vi "MainVI.vi"(0 "VISA resource name":refnum<visa-resource-name>="COM11", 1 "baud rate":u32=115200, 2 "data bits":u16=8 min=5 max=8 step=1, 3 "parity":u16(ring) items=["None", "Odd", "Even", "Mark", "Space"], 4 "stop bits":u16(ring)=10 items=["1.0"=10, "1.5"=15, "2.0"=20], 6 "read":bool=TRUE, 7 "flow control":u16(ring) items=["None"=0, "XON/XOFF"=1, "RTS/CTS"=2, "DTR/DSR"=4]) -> (9 "read string":string, 10 "bytes read":u32)   [LabVIEW 2017]
doc: "The Basic Serial Read and Write example performs a Serial Port Read, a Serial Port Write, or a combination of these actions. The user selects the actions (read or write) on the front panel. If both are selected, the VI will write the data first, read data, and then close the VISA session that is opened to the port. This VI will wait until the specified number of bytes is received at the port. Only the number of bytes specified will be read.\n\nINSTRUCTIONS:\n1) Select the serial resource and configuration parameters (baud rate, data bits, parity, stop bits, flow control).\n2) Select the operations to be performed. \n3) Connect the serial port to your device. If no device is available, perform a loopback test by doing one of the following. Short pins 2 and 3 on a RS-232 cable or short pin 4 to pin 8 and pin 5 to pin 9 on a RS-485/422 cable. \n4) Run the VI to see the data read. (The \"read string\" will match the \"string to write\" if a loopback test was performed.)\n\nNote: The parameters set for the serial port must match the parameters of the connected instrument or device. In this example, the bytes to read parameter specifies the number of bytes that the serial port reads. If there were more bytes at the port than the number specified in bytes to read, those bytes would not be read. Also, if you specify to read more bytes than the number of bytes actually read, you might receive a timeout error message.\n\nOn the block diagram, the Configure Serial Port VI sets the configuration parameters. The front panel displays the controls used to configure the basic parameters, such as baud rate, data bits, and parity. Constants configure the other parameters the user probably does not need set. After the VISA Configure Serial Port VI opens the VISA session and configures the port, the VI passes the VISA resource name to other VIs that perform operations on that VISA resource. The VISA Write function sends a command to the serial device and the VISA Read function returns data based on the command. The VISA Close function then closes the reference to the serial device. It is important to close the reference; otherwise communication through with that port through protocols other than VISA might not be possible."
uses:
  <vilib>/ErrorRing/Error Ring.xnode
panel:
  in  "file path (dialog if empty)":path
  in  "Tab Control":enum32{"Main", "Terminal", "Connect"}(tab)=enum."Terminal"
  out "Waveform Chart 4":dbl(graph)
  out "Waveform Chart 3":dbl(graph)
  out "Waveform Chart 2":dbl(graph)
  out "Waveform Chart":dbl(graph)
  in  "DTC":bool
  in  "Engine load":bool
  in  "Coolant temp.":bool
  in  "Engine RPM":bool
  in  "Speed":bool
  in  "Save to file":bool
  in  "Repeat":bool
  out "Return Count":u32
  in  "write":bool
  in  "string to write":string="ATZ"
  in  "Connect":bool
  in  "wbc":dbl=4.0
  out "Succses":u32
  in  "delay before read (ms)":u32=265
  out "Status":bool
  out "error out":errorcluster
  in  "stop":bool
  in  "Cancel Button":bool
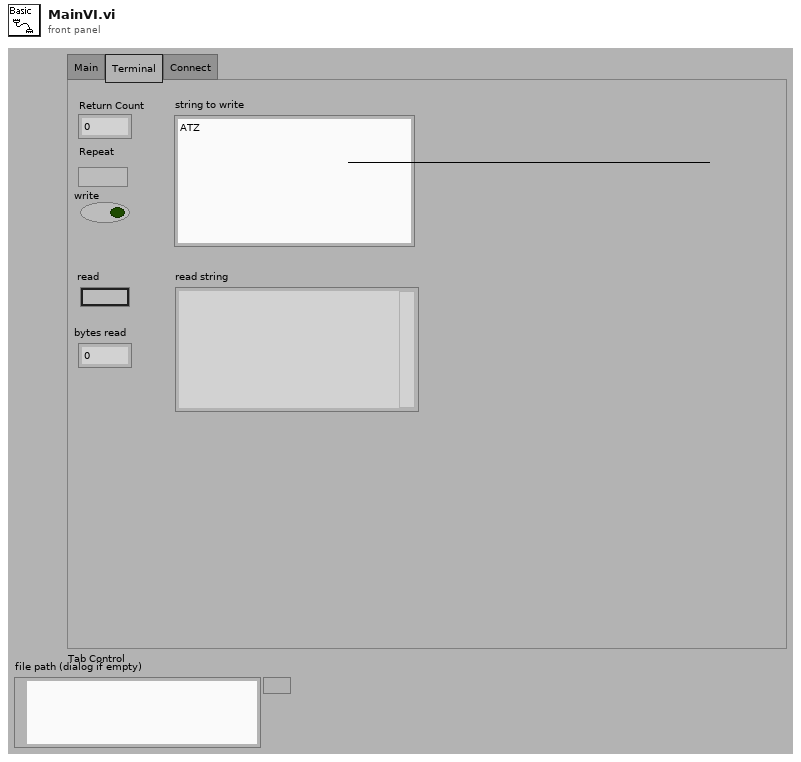
[diagram p1: front panel]
types:
  T1 = enum16{"open", "replace", "create", "open or create", "replace or create", "replace or create with confirmation"}
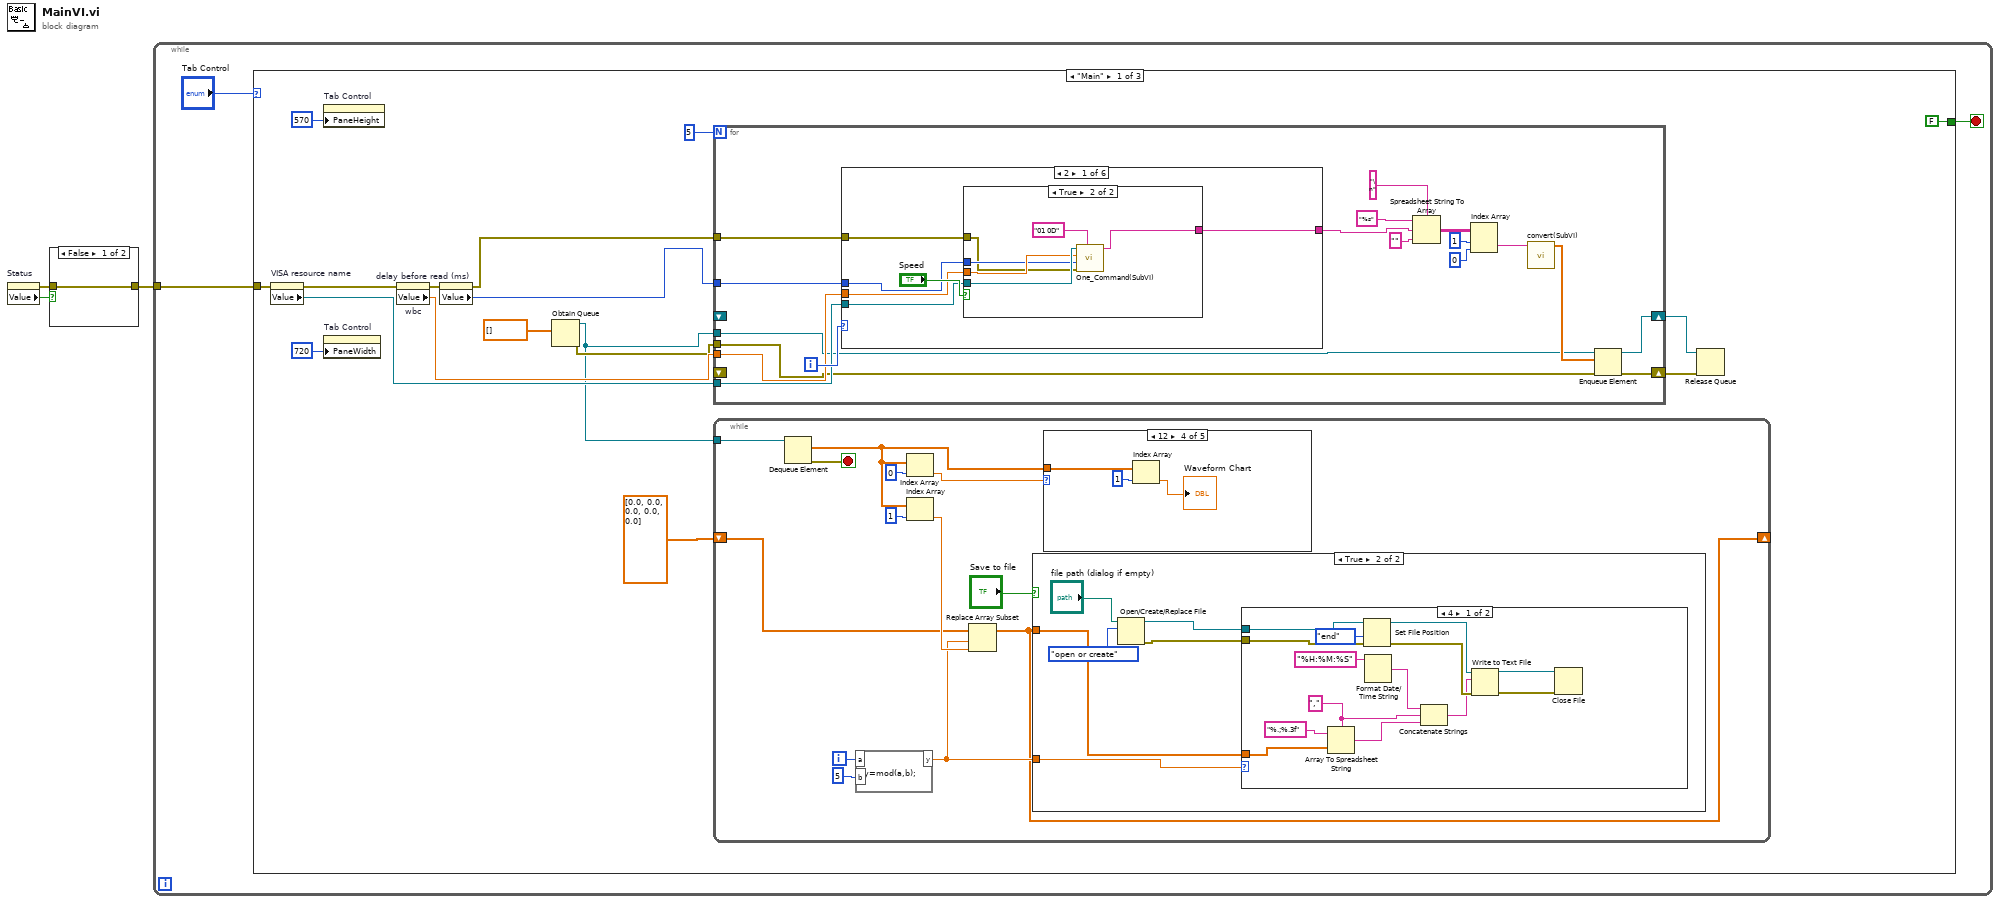
[diagram p0: block diagram]
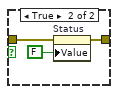
[diagram p2: hidden frame]
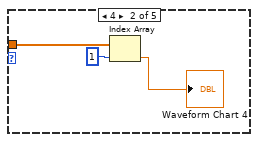
[diagram p6: hidden frame]
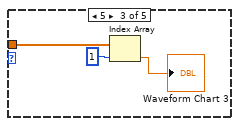
[diagram p7: hidden frame]
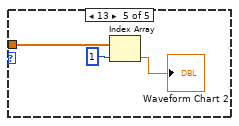
[diagram p8: hidden frame]
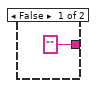
[diagram p9: hidden frame]
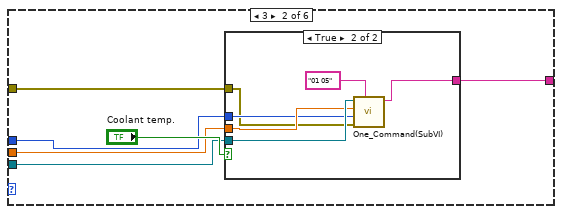
[diagram p10: hidden frame]
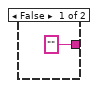
[diagram p11: hidden frame]
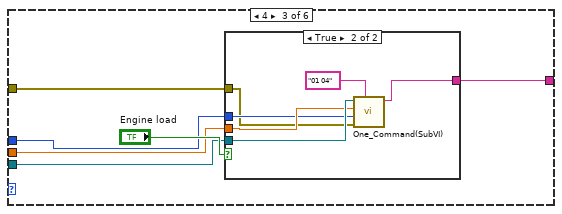
[diagram p12: hidden frame]
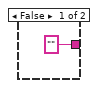
[diagram p13: hidden frame]
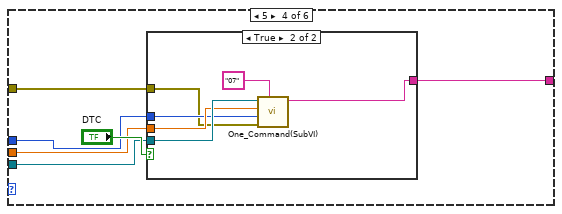
[diagram p14: hidden frame]
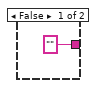
[diagram p15: hidden frame]
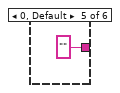
[diagram p16: hidden frame]
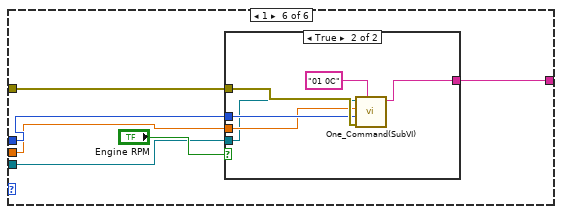
[diagram p17: hidden frame]
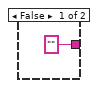
[diagram p18: hidden frame]
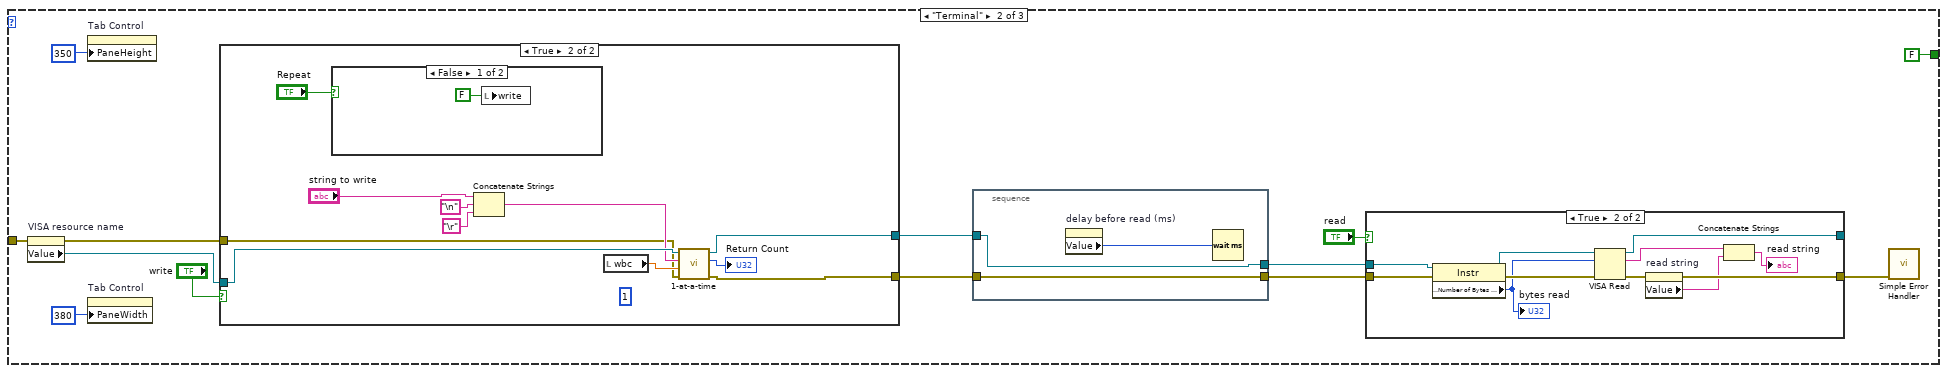
[diagram p19: hidden frame]
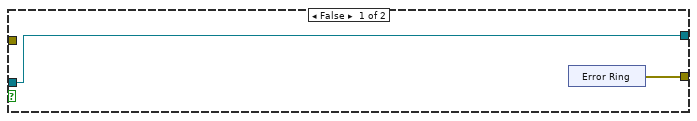
[diagram p20: hidden frame]
diagram:
  n1 = property on="Status" class="Bool (strict)"() -> (error out=w3:errorcluster, "Value"=w2:bool)  [unwired: 2 in, 1 out]
  n2 = case shown="False" w2 {
    tunnel: [w4 w7] -> w1
    tunnel: w3 -> [w4 w5]
    frame False {
    }
    frame True {
      n3 = property on="Status" class="Bool (strict)"(error in=w5, "Value"=FALSE) -> (error out=w7:errorcluster)  [unwired: 1 in, 1 out]
    }
  }
  n4 = while {
    tunnel: w1 -> [w8]
    stop <- w9 stop-if-true
    n5 = case shown="\"Main\"" "Tab Control" {
      tunnel: [FALSE FALSE "Cancel Button"] -> w9
      tunnel: w8 -> [w23 w157 w201]
      frame "Main" {
        n6 = property on="VISA resource name" class="VISAName"(error in=w23) -> (error out=w22:errorcluster, "Value"=w19:refnum<visa-resource-name>)  [unwired: 1 in, 1 out]
        n7 = property on="Tab Control" class="TabCtl (strict)"("PaneHeight"=570) -> ()  [unwired: 2 in, 2 out]
        n8 = property on="Tab Control" class="TabCtl (strict)"("PaneWidth"=720) -> ()  [unwired: 2 in, 2 out]
        n9 = property on="wbc" class="DigNum (strict)"(error in=w22) -> (error out=w21:errorcluster, "Value"=w18:dbl)  [unwired: 1 in, 1 out]
        n10 = property on="delay before read (ms)" class="DigNum (strict)"(error in=w21) -> (error out=w20:errorcluster, "Value"=w17:u32)  [unwired: 1 in, 1 out]
        n11 = Obtain Queue(element data type=dbl[] []) -> (queue out=w12:refnum<queue>, error out=w15:errorcluster)  [unwired: 4 in, 1 out]
        n12 = for {
          N: 5 -> [_]
          tunnel: w20 -> [w89]
          tunnel: w19 -> [w86]
          tunnel: w18 -> [w87]
          tunnel: w17 -> [w88]
          tunnel: w12 -> [w76]
          tunnel: w15 -> [w75]
          shift-right: [w74] -> w14
          shift-left: _ -> [_]
          shift-right: [w73] -> w13
          shift-left: _ -> [_]
          i -> [w90]
          n13 = case shown="2" w90 {
            tunnel: w89 -> [w95 w108 w121 w134 _ w148]
            tunnel: w88 -> [w92 w105 w118 w131 _ w147]
            tunnel: w87 -> [w93 w106 w119 w132 _ w146]
            tunnel: w86 -> [w94 w107 w120 w133 _ w145]
            tunnel: [w91 w104 w117 w130 "" w144] -> w82
            frame 2 {
              n14 = case shown="True" "Speed" {
                tunnel: w95 -> [_ w100]
                tunnel: w94 -> [_ w103]
                tunnel: w93 -> [_ w102]
                tunnel: w92 -> [_ w101]
                tunnel: ["" w98] -> w91
                frame False {
                }
                frame True {
                  n15 = call "One_Command(SubVI).vi"("string to write"="01 0D", "error in (no error)"=w100, "delay before read (ms)"=w101, "wbc"=w102, "VISA resource name"=w103) -> ("read string"=w98:string)  [unwired: 5 in, 1 out]
                }
              }
            }
            frame 3 {
              n16 = case shown="True" "Coolant temp." {
                tunnel: w108 -> [_ w113]
                tunnel: w107 -> [_ w116]
                tunnel: w106 -> [_ w115]
                tunnel: w105 -> [_ w114]
                tunnel: ["" w111] -> w104
                frame False {
                }
                frame True {
                  n17 = call "One_Command(SubVI).vi"("string to write"="01 05", "error in (no error)"=w113, "delay before read (ms)"=w114, "wbc"=w115, "VISA resource name"=w116) -> ("read string"=w111:string)  [unwired: 5 in, 1 out]
                }
              }
            }
            frame 4 {
              n18 = case shown="True" "Engine load" {
                tunnel: w121 -> [_ w126]
                tunnel: w120 -> [_ w129]
                tunnel: w119 -> [_ w128]
                tunnel: w118 -> [_ w127]
                tunnel: ["" w124] -> w117
                frame False {
                }
                frame True {
                  n19 = call "One_Command(SubVI).vi"("string to write"="01 04", "error in (no error)"=w126, "delay before read (ms)"=w127, "wbc"=w128, "VISA resource name"=w129) -> ("read string"=w124:string)  [unwired: 5 in, 1 out]
                }
              }
            }
            frame 5 {
              n20 = case shown="True" "DTC" {
                tunnel: w134 -> [_ w138]
                tunnel: w133 -> [_ w141]
                tunnel: w132 -> [_ w140]
                tunnel: w131 -> [_ w139]
                tunnel: ["" w137] -> w130
                frame False {
                }
                frame True {
                  n21 = call "One_Command(SubVI).vi"("string to write"="07", "error in (no error)"=w138, "delay before read (ms)"=w139, "wbc"=w140, "VISA resource name"=w141) -> ("read string"=w137:string)  [unwired: 5 in, 1 out]
                }
              }
            }
            frame 0, Default {
            }
            frame 1 {
              n22 = case shown="True" "Engine RPM" {
                tunnel: w148 -> [_ w156]
                tunnel: w147 -> [_ w155]
                tunnel: w146 -> [_ w154]
                tunnel: w145 -> [_ w153]
                tunnel: ["" w151] -> w144
                frame False {
                }
                frame True {
                  n23 = call "One_Command(SubVI).vi"("string to write"="01 0C", "error in (no error)"=w156, "delay before read (ms)"=w155, "wbc"=w154, "VISA resource name"=w153) -> ("read string"=w151:string)  [unwired: 5 in, 1 out]
                }
              }
            }
          }
          n24 = Spreadsheet String To Array(delimiter (Tab)="\n", format string="%s" ("spreadsheet string"), spreadsheet string=w82, array type (2D Dbl)="") -> (array=w80:string[][])
          n25 = Index Array(array=w80, index (row)=1, index (col)=0 ("disabled index (col)")) -> (element=w78:string)
          n26 = call "convert(SubVI).vi"("String in"=w78) -> ("Array"=w77:dbl[])  [unwired: 10 in]
          n27 = Enqueue Element(queue=w76, element=w77, error in (no error)=w75) -> (queue out=w74:refnum<queue>, error out=w73:errorcluster)  [unwired: 1 in, 1 out]
        }
        n28 = while {
          tunnel: w12 -> [w40]
          shift-right: [w29] -> _
          shift-left: dbl[] [0.0, 0.0, 0.0, 0.0, 0.0] -> [w31]
          i -> [w36]
          stop <- w39 stop-if-true
          n29 = Dequeue Element(queue=w40) -> (element=w33:dbl[], error out=w39:errorcluster)  [unwired: 2 in, 2 out]
          n30 = formula code="y=mod(a,b);"("a"=w36, "b"=5 ("input variable")) -> ("y"=w30:dbl)
          n31 = Index Array(array=w33, index=0) -> (element=w37:dbl)
          n32 = Index Array(array=w33, index=1) -> (element=w32:dbl)
          n33 = Replace Array Subset(array=w31, new element=w32, index=w30) -> (w29:dbl[])
          n34 = case shown="True" "Save to file" {
            tunnel: w30 -> [_ w46]
            tunnel: w29 -> [_ w45]
            frame False {
            }
            frame True {
              n35 = Open/Create/Replace File(file path (use dialog)="file path (dialog if empty)", operation (0:open)=T1."open or create") -> (refnum out=w43:refnum<file>, error out=w42:errorcluster)  [unwired: 4 in, 1 out]
              n36 = case shown="4" w46 {
                tunnel: w45 -> [w59 _]
                tunnel: w43 -> [w55 _]
                tunnel: w42 -> [w54 _]
                frame 4 {
                  w47 = "," ("delimiter (Tab)")
                  n37 = Array To Spreadsheet String(delimiter (Tab)=w47, array=w59, 3:"%.;%.3f" ("format string")) -> (spreadsheet string=w57:string)
                  n38 = Set File Position(refnum=w55, from (0:start)=enum16{"start", "end", "current"}."end", error in=w54) -> (refnum out=w53:refnum<file>, error out=w52:errorcluster)  [unwired: 1 in]
                  n39 = Format Date/Time String(time format string (%c)="%H:%M:%S") -> (date/time string=w58:string)  [unwired: 2 in]
                  n40 = Concatenate Strings(w58, w47, w57) -> (w51:string)
                  n41 = Write to Text File(file (use dialog)=w53, text=w51, error in=w52) -> (refnum out=w50:refnum<file>, error out=w49:errorcluster)  [unwired: 1 in, 1 out]
                  n42 = Close File(refnum=w50, error in=w49) -> ()  [unwired: 2 out]
                }
                frame Default {
                }
              }
            }
          }
          n43 = case shown="12" w37 {
            tunnel: w33 -> [_ w62 w65 w68 w71]
            frame Default {
            }
            frame 4 {
              n44 = Index Array(array=w62, index=1) -> (element=→"Waveform Chart 4":dbl)
            }
            frame 5 {
              n45 = Index Array(array=w65, index=1) -> (element=→"Waveform Chart 3":dbl)
            }
            frame 12 {
              n46 = Index Array(array=w68, index=1) -> (element=→"Waveform Chart":dbl)
            }
            frame 13 {
              n47 = Index Array(array=w71, index=1) -> (element=→"Waveform Chart 2":dbl)
            }
          }
        }
        n48 = Release Queue(queue=w14, error in (no error)=w13) -> ()  [unwired: 1 in, 3 out]
      }
      frame "Terminal" {
        n49 = property on="VISA resource name" class="VISAName"(error in=w157) -> (error out=w158:errorcluster, "Value"=w159:refnum<visa-resource-name>)  [unwired: 1 in, 1 out]
        n50 = property on="Tab Control" class="TabCtl (strict)"("PaneHeight"=350) -> ()  [unwired: 2 in, 2 out]
        n51 = property on="Tab Control" class="TabCtl (strict)"("PaneWidth"=380) -> ()  [unwired: 2 in, 2 out]
        n52 = case shown="True" "write" {
          tunnel: [w173 w186] -> w166
          tunnel: w159 -> [w174 w185]
          tunnel: [w174 w184] -> w165
          tunnel: w158 -> [_ w176]
          frame False {
            n53 = xnode "Error Ring"() -> ("error out"=w173:errorcluster)
          }
          frame True {
            (unwired) u32 1 ("Wait Between Characters(ms)")
            n54 = case shown="False" "Repeat" {
              frame False {
                n55 = local write "write"(FALSE) -> ()
              }
              frame True {
              }
            }
            n56 = Concatenate Strings("string to write", "\n", "\r") -> (w181:string)
            n57 = local read "wbc"() -> (w177:dbl)
            n58 = call "1-at-a-time.vi"("error in (no error)"=w176, "Wait Between Characters(ms)"=w177, "write buffer"=w181, "VISA resource name"=w185) -> ("error out"=w186:errorcluster, "Return Count"=→"Return Count":u32, "VISA resource name out"=w184:refnum<visa-resource-name>)  [unwired: 5 in]
          }
        }
        n59 = stacked-sequence {
          tunnel: w166 -> [w172]
          tunnel: [w172] -> w163
          tunnel: w165 -> [w171]
          tunnel: [w171] -> w164
          frame #0 {
            n60 = property on="delay before read (ms)" class="DigNum (strict)"() -> ("Value"=w170:u32)  [unwired: 2 in, 2 out]
            n61 = Wait (ms)(milliseconds to wait=w170) -> ()  [unwired: 1 out]
          }
        }
        n62 = case shown="True" "read" {
          tunnel: w163 -> [w189 w197]
          tunnel: [w189 w191] -> w169
          tunnel: [w188 w200] -> _
          tunnel: w164 -> [w188 w199]
          frame False {
          }
          frame True {
            n63 = property class="Instr"(reference=w199, error in=w197) -> (reference out=w198:refnum<visa-resource-name>, error out=w196:errorcluster, "Serial Settings:Number of Bytes at Serial Port"=w195:u32)
            "bytes read" <- w195
            n64 = VISA Read(VISA resource name=w198, byte count=w195, error in (no error)=w196) -> (VISA resource name out=w200:refnum<visa-resource-name>, read buffer=w194:string, error out=w192:errorcluster)  [unwired: 1 out]
            n65 = property on="read string" class="Str"(error in=w192) -> (error out=w191:errorcluster, "Value"=w190:string)  [unwired: 1 in, 1 out]
            n66 = Concatenate Strings(w194, w190) -> (→"read string":string)
          }
        }
        n67 = call <vilib>:"Simple Error Handler.vi"("error in (no error)"=w169) -> ()  [unwired: 4 in, 5 out]
      }
      frame "Connect", Default {
        n68 = property on="Tab Control" class="TabCtl (strict)"("PaneHeight"=400) -> ()  [unwired: 2 in, 2 out]
        n69 = case shown="True" "Connect" {
          tunnel: w201 -> [_ w211]
          frame False {
          }
          frame True {
            n70 = while {
              tunnel: [w217] -> w213
              tunnel: w211 -> [w214]
              stop <- w216 stop-if-true
              n71 = call "Serial_Init(SubVI).vi"("VISA Refnum in"="VISA resource name", "wbc"="wbc", "delay before read (ms)"="delay before read (ms)", "baud rate"="baud rate", "error in (no error)"=w214, "data bits"="data bits", "parity"="parity", "stop bits"="stop bits", "flow control"="flow control") -> ("Success_out"=w215:i32, "error out"=w217:errorcluster)  [unwired: 8 in, 1 out]
              "Succses" <- w215
              n72 = Equal?(x=9, y=w215) -> (x = y?=w216:bool)
              "Status" <- w216
            }
            n73 = stacked-sequence {
              tunnel: w213 -> [w228]
              tunnel: [w227] -> w212
              frame #0 {
                n74 = Wait (ms)(milliseconds to wait=u32 1000 ("delay before read (ms) 2")) -> ()  [unwired: 1 out]
                n75 = property on="read string" class="Str"(error in=w228, "Value"="") -> (error out=w227:errorcluster)  [unwired: 1 in, 1 out]
              }
            }
            "error out" <- w212
            n76 = call <vilib>:"Simple Error Handler.vi"("error in (no error)"=w212) -> ()  [unwired: 4 in, 5 out]
          }
        }
        n77 = property on="Tab Control" class="TabCtl (strict)"("PaneWidth"=470) -> ()  [unwired: 2 in, 2 out]
        n78 = case shown="False" "stop" {
          frame False {
          }
          frame True {
            n79 = property on="VISA resource name" class="VISAName"() -> ("Value"=w210:refnum<visa-resource-name>)  [unwired: 2 in, 2 out]
            n80 = VISA Close(VISA resource name=w210) -> (error out=w208:errorcluster)  [unwired: 1 in]
            n81 = property on="Status" class="Bool (strict)"(error in=w208, "Value"=FALSE) -> (error out=w207:errorcluster)  [unwired: 1 in, 1 out]
            n82 = call <vilib>:"Simple Error Handler.vi"("error in (no error)"=w207) -> ()  [unwired: 4 in, 5 out]
          }
        }
      }
    }
  }
